vi "Execute Measurement.vi"(0 "Measurement Client Wrapper":refnum<class "Measurement Client Wrapper.lvclass">, 11 "error in":errorcluster) -> (4 "Measurement Client Wrapper out":refnum<class "Measurement Client Wrapper.lvclass">, 15 "error out":errorcluster)   [LabVIEW 2020, in "Measurement Client Wrapper.lvclass"]
uses:
  Measurement Client Wrapper.lvclass
  Measurement Client Wrapper.lvclass/Measurement Client Wrapper.ctl
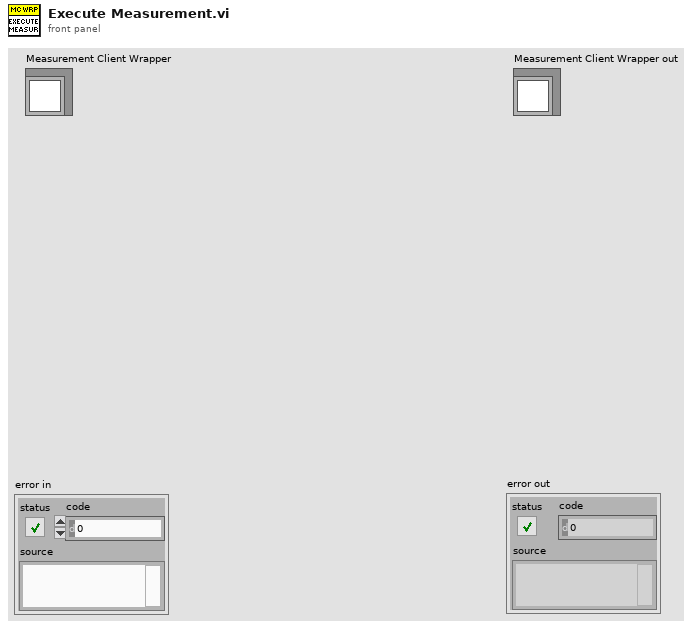
[diagram p1: front panel]
types:
  T1 = typedef "Measurement Client Wrapper.lvclass/Measurement Parameter Details.ctl" = cluster{"Name":string, "Parent":string, "ProtobufID":i32, "Measurement DataType":T2, "Array Dimension":i32}
  T2 = typedef "Measurement Client Wrapper.lvclass/Measurement DataType.ctl" = enum16{"UNSPECIFIED", "BOOL", "DOUBLE", "FLOAT", "INT32", "INT64", "STRING", "UINT32", "UINT64"}
  T3 = typedef "Measurement Client Wrapper.lvclass/Control UI MetaData.ctl" = cluster{"Name":string, "Parent":string, "LabVIEW DataType":T4, "Measurement DataType":T2, "Value":variant, "Array Dimension":i32}
  T4 = typedef "NI_Data Type.lvlib/Data Type.ctl" = enum8{"Invalid Type", "Void", "I8", "I16", "I32", "I64", "U8", "U16", "U32", "U64", "Single Float", "Double Float", "Extended Float", "Single Complex", "Double Complex", "Extended Complex", "Enum U8", "Enum U16", "Enum U32", "Enum U64", "Single Float With Unit", "Double Float With Unit", "Extended Float With Unit", "Single Complex with Unit", "Double Complex with Unit", "Extended Complex with Unit", "Boolean", "String", "Path", "Picture", "Tag", "Array", "Cluster", "Variant", "LV Variant", "Waveform", "Timestamp", "Digital Waveform", "Digital Data", "ExpressData", "Refnum", "External Data", "VI", "Poly VI", "LabVIEW Class Instance", "Fixed Point", "Set Collection", "Map Collection"}
  T5 = cluster{"Measurement DataType":T2, "Array Dimension":i32, "Value":variant}
  T6 = cluster{"Measurement DataType":T2, "Array Dimension":i32, "Data":variant}[]
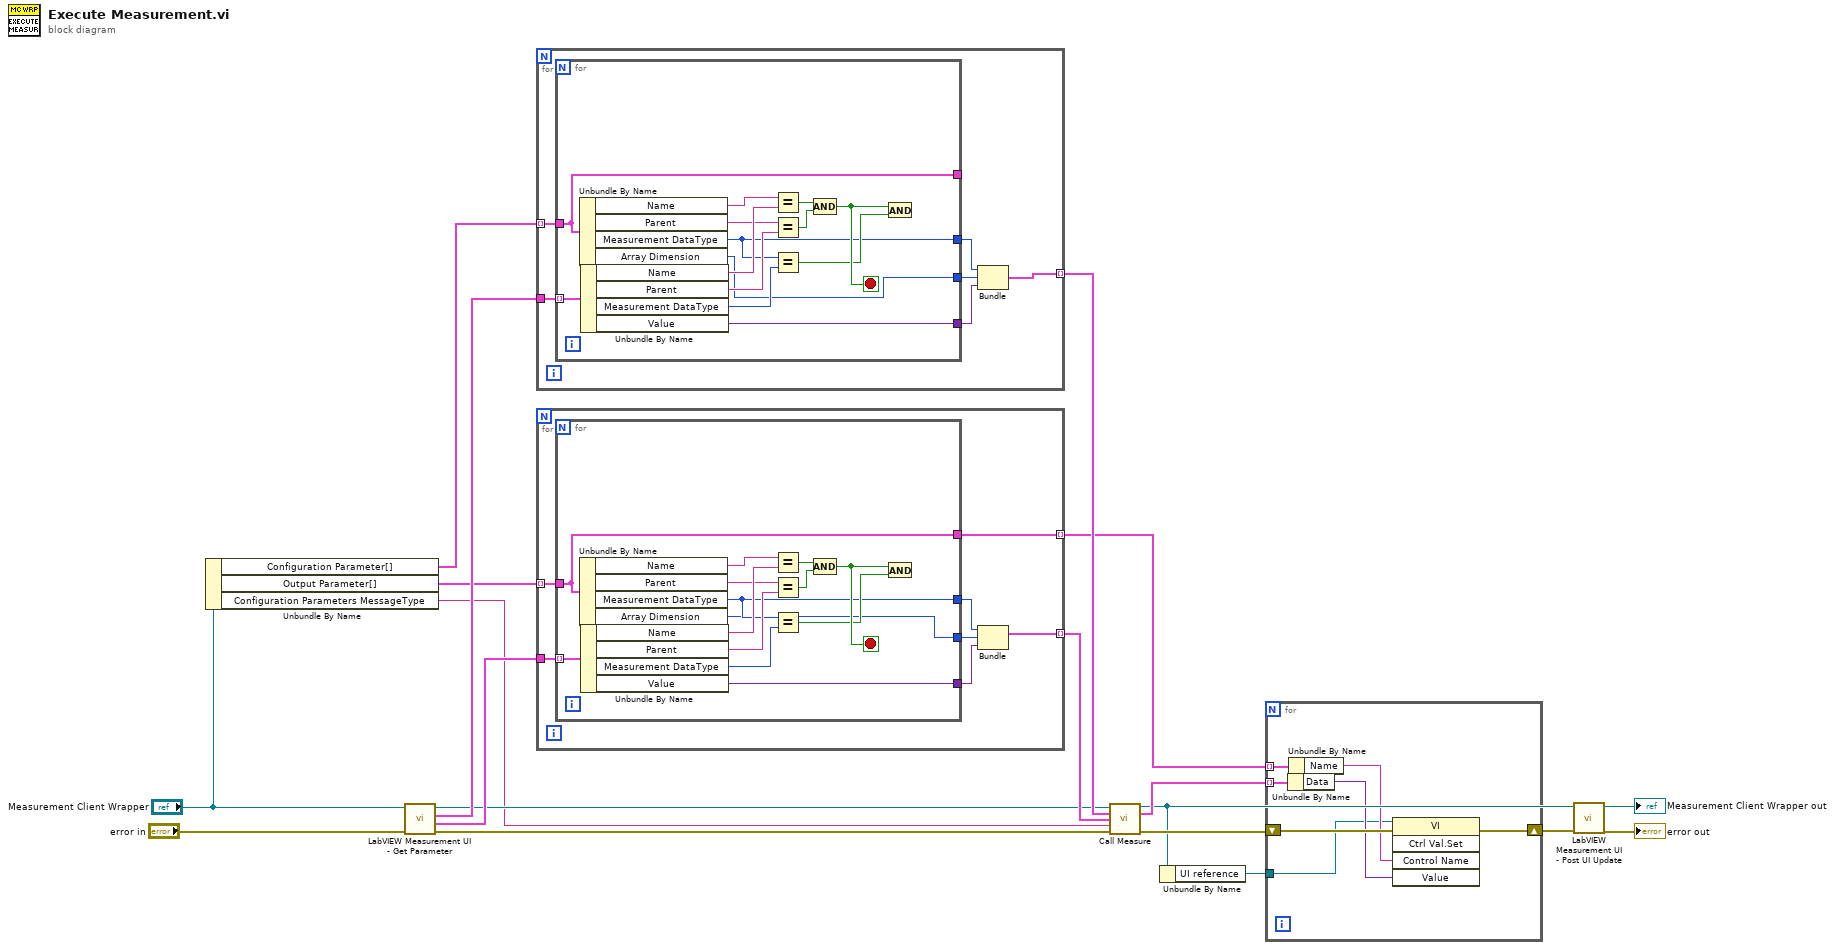
[diagram p0: block diagram]
diagram:
  n1 = Unbundle By Name("Measurement Client Wrapper") -> ("Configuration Parameter[]"=w3:T1[], "Output Parameter[]"=w8:T1[], "Configuration Parameters MessageType"=w1:string)
  n2 = call "LabVIEW Measurement UI - Get Parameter.vi"("error in"="error in", "Measurement Client Wrapper in"="Measurement Client Wrapper") -> ("error out"=w18:errorcluster, "UI Indicator Details[]"=w15:T3[], "UI Control Details[]"=w17:T3[], "Measurement Client Wrapper"=w10:refnum<class "Measurement Client Wrapper.lvclass">)  [unwired: 6 in]
  n3 = for {
    tunnel: w3 -> [w24] mode=indexing
    tunnel: w17 -> [w25]
    tunnel: [w21] -> w16 mode=indexing
    n4 = for {
      tunnel: w25 -> [w39] mode=indexing
      tunnel: w24 -> [w29]
      tunnel: [w29] -> _
      tunnel: [w28] -> w22
      tunnel: [w27] -> w23
      tunnel: [w26] -> w20
      stop <- w33 stop-if-true
      n5 = Unbundle By Name(w29) -> ("Name"=w31:string, "Parent"=w30:string, "Measurement DataType"=w27:T2, "Array Dimension"=w26:i32)
      n6 = Unbundle By Name(w39) -> ("Name"=w38:string, "Parent"=w37:string, "Measurement DataType"=w36:T2, "Value"=w28:variant)
      n7 = Equal?(x=w31, y=w38) -> (x = y?=w35:bool)
      n8 = Equal?(x=w30, y=w37) -> (x = y?=w34:bool)
      n9 = Equal?(x=w27, y=w36) -> (x = y?=w32:bool)
      n10 = Compound Arithmetic op=AND(w35, w34) -> (w33:bool)
      n11 = And(x=w33, y=w32) -> ()  [unwired: 1 out]
    }
    n12 = Bundle("Measurement DataType"=w23, "Array Dimension"=w20, "Value"=w22) -> (w21:T5)  [unwired: 1 in]
  }
  n13 = for {
    tunnel: w8 -> [w45] mode=indexing
    tunnel: w15 -> [w46]
    tunnel: [w42] -> w14 mode=indexing
    tunnel: [w41] -> w12 mode=indexing
    n14 = for {
      tunnel: w46 -> [w60] mode=indexing
      tunnel: w45 -> [w50]
      tunnel: [w50] -> w41
      tunnel: [w49] -> w43
      tunnel: [w48] -> w44
      tunnel: [w47] -> w40
      stop <- w54 stop-if-true
      n15 = Unbundle By Name(w50) -> ("Name"=w52:string, "Parent"=w51:string, "Measurement DataType"=w48:T2, "Array Dimension"=w47:i32)
      n16 = Unbundle By Name(w60) -> ("Name"=w59:string, "Parent"=w58:string, "Measurement DataType"=w57:T2, "Value"=w49:variant)
      n17 = Equal?(x=w52, y=w59) -> (x = y?=w56:bool)
      n18 = Equal?(x=w51, y=w58) -> (x = y?=w55:bool)
      n19 = Equal?(x=w48, y=w57) -> (x = y?=w53:bool)
      n20 = Compound Arithmetic op=AND(w56, w55) -> (w54:bool)
      n21 = And(x=w54, y=w53) -> ()  [unwired: 1 out]
    }
    n22 = Bundle("Measurement DataType"=w44, "Array Dimension"=w40, "Value"=w43) -> (w42:T5)  [unwired: 1 in]
  }
  n23 = call "Call Measure.vi"("Measurement Client Wrapper in"=w10, "Config Data"=w16, "Expected Output Format"=w14, "ConfigurationParametersMessagetype"=w1, "error in (no error)"=w18) -> ("Measurement Client Wrapper out"=w6:refnum<class "Measurement Client Wrapper.lvclass">, "Output Data"=w11:T6, "error out"=w13:errorcluster)  [unwired: 8 in]
  n24 = Unbundle By Name(w6) -> ("UI reference"=w9:refnum<vi>)
  n25 = for {
    shift-right: [w66] -> w7
    shift-left: w13 -> [w67]
    tunnel: w12 -> [w64] mode=indexing
    tunnel: w11 -> [w63] mode=indexing
    tunnel: w9 -> [w61]
    n26 = Unbundle By Name(w63) -> ("Data"=w62:variant)
    n27 = Unbundle By Name(w64) -> ("Name"=w65:string)
    n28 = invoke class="VI" method="Ctrl Val.Set"(reference=w61, error in=w67, "Control Name"=w65, "Value"=w62) -> (error out=w66:errorcluster)  [unwired: 1 in, 4 out]
  }
  n29 = call "LabVIEW Measurement UI - Post UI Update.vi"("error in"=w7, "Measurement Client Wrapper in"=w6) -> ("error out"=→"error out":errorcluster, "Measurement Client Wrapper"=→"Measurement Client Wrapper out":refnum<class "Measurement Client Wrapper.lvclass">)  [unwired: 8 in]
